vi "Read Range.vi"(8 "error in (no error)":errorcluster, 11 "Scanner.lvclass in":refnum<class "Scanner.lvclass">) -> (0 "error out":errorcluster, 1 "Range":T1, 2 "# Points":u32, 3 "Scanner.lvclass out":refnum<class "Scanner.lvclass">, 4 "Return to start?":bool, 5 "Scanning Up?":bool)   [LabVIEW 2009, in "Scanner.lvclass"]
doc: "Return the Range of this Scanner."
uses:
  Scanner.lvclass
  Range.ctl
  Scanner.lvclass/Scanner.ctl
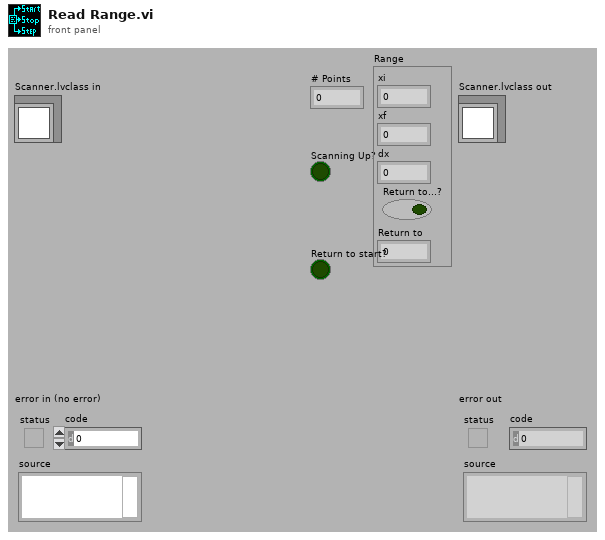
[diagram p1: front panel]
types:
  T1 = typedef "Scanner.lvclass/Range.ctl" = cluster{"xi":dbl, "xf":dbl, "dx":dbl, "Return to...?":bool, "Return to":dbl}
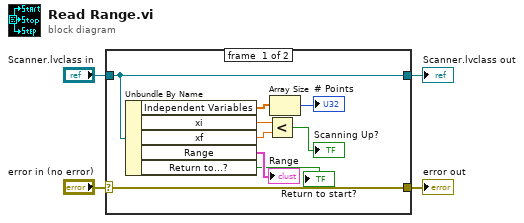
[diagram p0: block diagram]
diagram:
  n1 = case shown="No Error" "error in (no error)" {
    selector: "error in (no error)" -> [w13 w14]
    tunnel: [w13 w14] -> w3
    tunnel: [w12 w15] -> w1
    tunnel: "Scanner.lvclass in" -> [w12 w15]
    frame #0 {
      n2 = Unbundle By Name(w12) -> ("Independent Variables"=w11:dbl[], "xi"=w9:dbl, "xf"=w8:dbl, "Range"=→"Range":T1, "Return to...?"=→"Return to start?":bool)
      n3 = Less?(x=w9, y=w8) -> (x < y?=→"Scanning Up?":bool)
      n4 = Array Size(array=w11) -> (size(s)=→"# Points":i32)
    }
    frame #1 {
    }
  }
  "error out" <- w3
  "Scanner.lvclass out" <- w1
